vi "NCS_RxTxSetup.vi"(0 "IVI Refnum in":refnum<k15>, 1 "Rx IQ Rate":dbl, 2 "Start Trigger Time":T1={"whole seconds"=1, "fractional seconds"=0.0}, 3 "Configuration:Enabled Channels":string, 4 "Tx IQ Rate":dbl, 5 "Tx Gain":dbl, 6 "Tx carrier frequency [Hz]":dbl, 8 "Rx Gain":dbl, 9 "Tx active antenna":string, 10 "Rx carrier frequency [Hz]":dbl, 11 "Active Channel":string, 12 "Rx Active Antenna":string, 14 "Active Channel 2":string) -> (18 "session handle out":refnum<k15>, 20 "IVI Refnum out":refnum<k15>, 21 "Coerced Rx IQ Rate":dbl, 22 "Bandwidth":dbl, 23 "Gain":dbl, 24 "Carrier Frequency":dbl, 25 "IQ Rate 2":dbl, 27 "error out":errorcluster)   [LabVIEW 2016]
uses:
  <instrlib>/niUSRP/niUSRP Timestamp.ctl
  <instrlib>/niUSRP/niUSRP Configure Time Start Trigger.vi
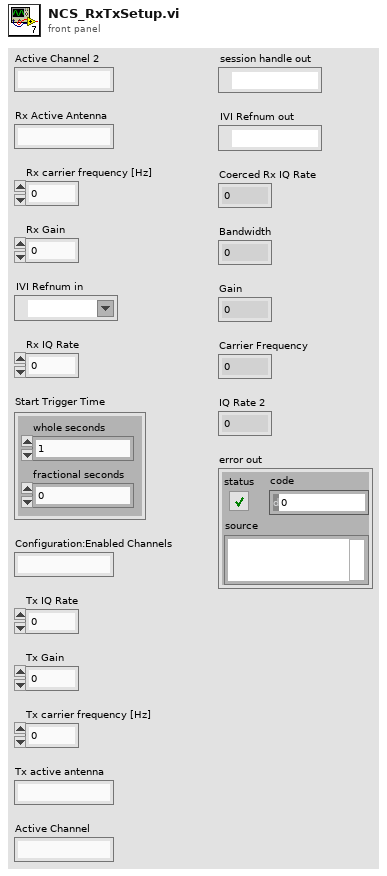
[diagram p1: front panel]
types:
  T1 = typedef "niUSRP Timestamp.ctl" = cluster{"whole seconds":u64, "fractional seconds":dbl}
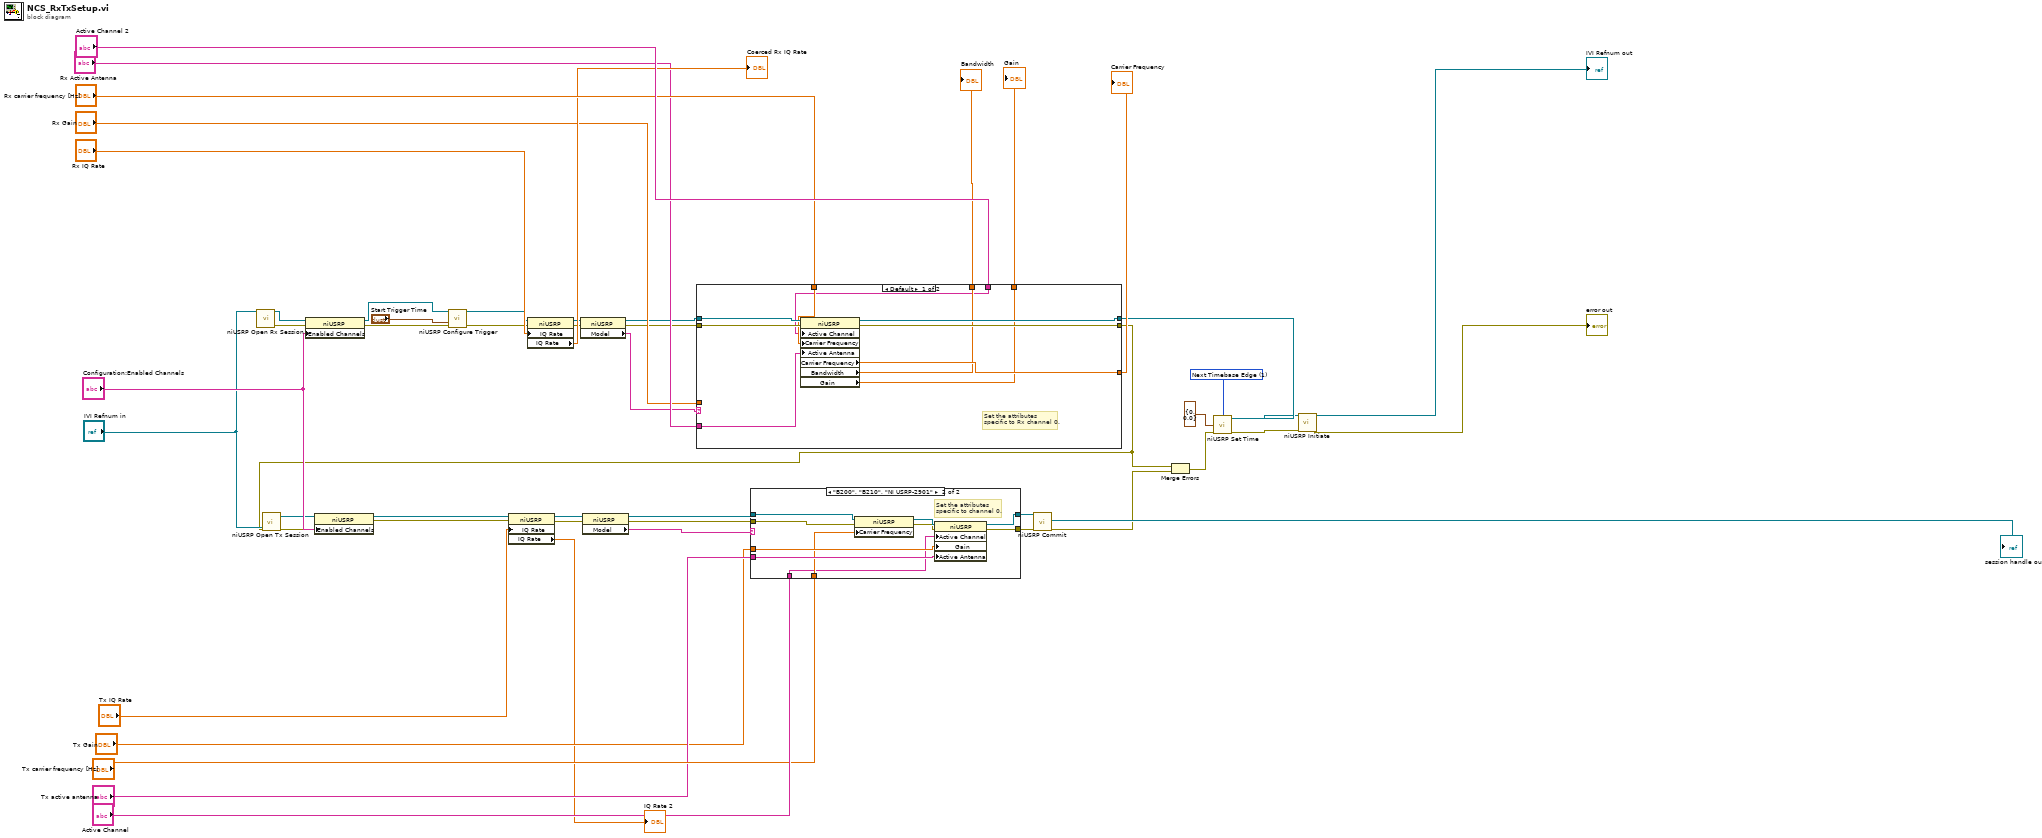
[diagram p0: block diagram]
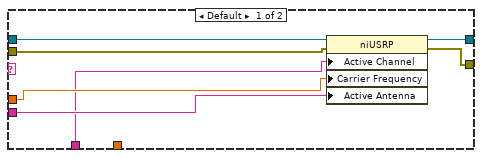
[diagram p2: hidden frame]
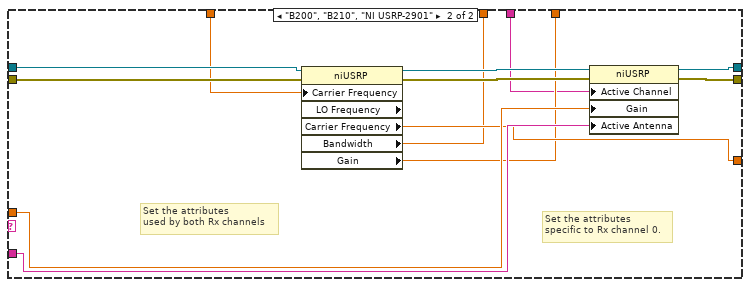
[diagram p3: hidden frame]
diagram:
  w10 = 1 items=["Now", "Next Timebase Edge"] ("apply timestamp")
  n1 = call <instrlib>:"niUSRP Open Rx Session.vi"("device names"="IVI Refnum in") -> ("session handle out"=w11:refnum<k15>, "error out"=w12:errorcluster)  [unwired: 13 in]
  n2 = property class="niUSRP"(reference=w11, error in=w12, "Enabled Channels"="Configuration:Enabled Channels") -> (reference out=w13:refnum<k15>, error out=w14:errorcluster)
  n3 = call-poly <instrlib>:"niUSRP Configure Trigger.vi"("session handle"=w13, "start trigger time"="Start Trigger Time", "error in (no error)"=w14) -> ("session handle out"=w17:refnum<k15>, "error out"=w18:errorcluster)  [unwired: 11 in]
  n4 = property class="niUSRP"(reference=w17, error in=w18, "IQ Rate"="Rx IQ Rate") -> (reference out=w21:refnum<k15>, error out=w20:errorcluster, "IQ Rate"=→"Coerced Rx IQ Rate":dbl)
  n5 = property class="niUSRP"(reference=w21, error in=w20) -> (reference out=w25:refnum<k15>, error out=w24:errorcluster, "Model"=w23:string)
  n6 = case shown="Default" w23 {
    tunnel: w24 -> [w61 w71]
    tunnel: w25 -> [w60 w72]
    tunnel: [w58 w68] -> w22
    tunnel: [w57 w67] -> w1
    tunnel: "Rx Gain" -> [_ w74]
    tunnel: "Rx Active Antenna" -> [w59 w73]
    tunnel: [w56 w66] -> w49
    tunnel: "Rx carrier frequency [Hz]" -> [w53 w65]
    tunnel: [w55 w64] -> w47
    tunnel: [w54 w63] -> w48
    tunnel: "Active Channel 2" -> [w52 w62]
    frame Default {
      # "Set the attributes \nspecific to Rx channel 0."
      n7 = property class="niUSRP"(reference=w60, error in=w61, "Active Channel"=w52, "Carrier Frequency"=w53, "Active Antenna"=w59) -> (reference out=w58:refnum<k15>, error out=w57:errorcluster, "Carrier Frequency"=w56:dbl, "Bandwidth"=w55:dbl, "Gain"=w54:dbl)
    }
    frame "B200", "B210", "NI USRP-2901" {
      # "Set the attributes \nused by both Rx channels"
      # "Set the attributes \nspecific to Rx channel 0."
      n8 = property class="niUSRP" props=["Carrier Frequency", "LO Frequency", "Carrier Frequency", "Bandwidth", "Gain"](reference=w72, error in=w71, "Carrier Frequency"=w65) -> (reference out=w70:refnum<k15>, error out=w69:errorcluster, "Carrier Frequency"=w66:dbl, "Bandwidth"=w64:dbl, "Gain"=w63:dbl)  [unwired: 1 out]
      n9 = property class="niUSRP"(reference=w70, error in=w69, "Active Channel"=w62, "Gain"=w74, "Active Antenna"=w73) -> (reference out=w68:refnum<k15>, error out=w67:errorcluster)
    }
  }
  "Carrier Frequency" <- w49
  "Gain" <- w48
  "Bandwidth" <- w47
  n10 = call <instrlib>:"niUSRP Open Tx Session.vi"("device names"="IVI Refnum in", "error in (no error)"=w1) -> ("session handle out"=w15:refnum<k15>, "error out"=w16:errorcluster)  [unwired: 12 in]
  n11 = property class="niUSRP"(reference=w15, error in=w16, "Enabled Channels"="Configuration:Enabled Channels") -> (reference out=w28:refnum<k15>, error out=w29:errorcluster)
  n12 = property class="niUSRP"(reference=w28, error in=w29, "IQ Rate"="Tx IQ Rate") -> (reference out=w34:refnum<k15>, error out=w33:errorcluster, "IQ Rate"=→"IQ Rate 2":dbl)
  n13 = property class="niUSRP"(reference=w34, error in=w33) -> (reference out=w32:refnum<k15>, error out=w31:errorcluster, "Model"=w35:string)
  n14 = case shown="\"B200\", \"B210\", \"NI USRP-2901\"" w35 {
    tunnel: "Tx Gain" -> [w76 w91]
    tunnel: "Tx active antenna" -> [w81 w90]
    tunnel: [w78 w85] -> w38
    tunnel: [w77 w84] -> w37
    tunnel: w31 -> [w80 w86]
    tunnel: w32 -> [w79 w89]
    tunnel: "Tx carrier frequency [Hz]" -> [_ w83]
    tunnel: "Active Channel" -> [w75 w82]
    frame Default {
      n15 = property class="niUSRP"(reference=w79, error in=w80, "Active Channel"=w75, "Carrier Frequency"=w76, "Active Antenna"=w81) -> (reference out=w78:refnum<k15>, error out=w77:errorcluster)
    }
    frame "B200", "B210", "NI USRP-2901" {
      # "Set the attributes \nspecific to channel 0."
      n16 = property class="niUSRP"(reference=w89, error in=w86, "Carrier Frequency"=w83) -> (reference out=w88:refnum<k15>, error out=w87:errorcluster)
      n17 = property class="niUSRP"(reference=w88, error in=w87, "Active Channel"=w82, "Gain"=w91, "Active Antenna"=w90) -> (reference out=w85:refnum<k15>, error out=w84:errorcluster)
    }
  }
  n18 = call <instrlib>:"niUSRP Commit.vi"("session handle"=w38, "error in (no error)"=w37) -> ("session handle out"=→"session handle out":refnum<k15>, "error out"=w3:errorcluster)  [unwired: 12 in]
  n19 = Merge Errors(w1, w3) -> (w8:errorcluster)
  n20 = call <instrlib>:"niUSRP Set Time.vi"("session handle"=w22, "apply timestamp"=w10, "timestamp"=T1 {"whole seconds"=0, "fractional seconds"=0.0}, "error in (no error)"=w8) -> ("session handle out"=w6:refnum<k15>, "error out"=w7:errorcluster)  [unwired: 10 in]
  n21 = call <instrlib>:"niUSRP Initiate.vi"("session handle"=w6, "error in (no error)"=w7) -> ("session handle out"=→"IVI Refnum out":refnum<k15>, "error out"=→"error out":errorcluster)  [unwired: 12 in]
